vi "hamamatsuReadSegment.vi"() -> ()   [LabVIEW 2017]
uses:
  globalDevices.vi
  globalUtilities.vi
panel:
  out "Frame Count":i32
  out "Numeric":i32
  out "error out":errorcluster {"code" format="%.0x"}
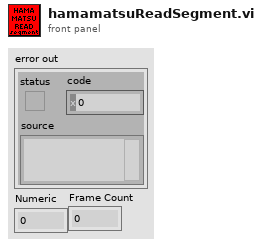
[diagram p1: front panel]
types:
  T1 = enum16{"open", "replace", "create", "open or create", "replace or create", "replace or create with confirmation"}
  T2 = enum16{"big-endian, network order", "native, host order", "little-endian"}
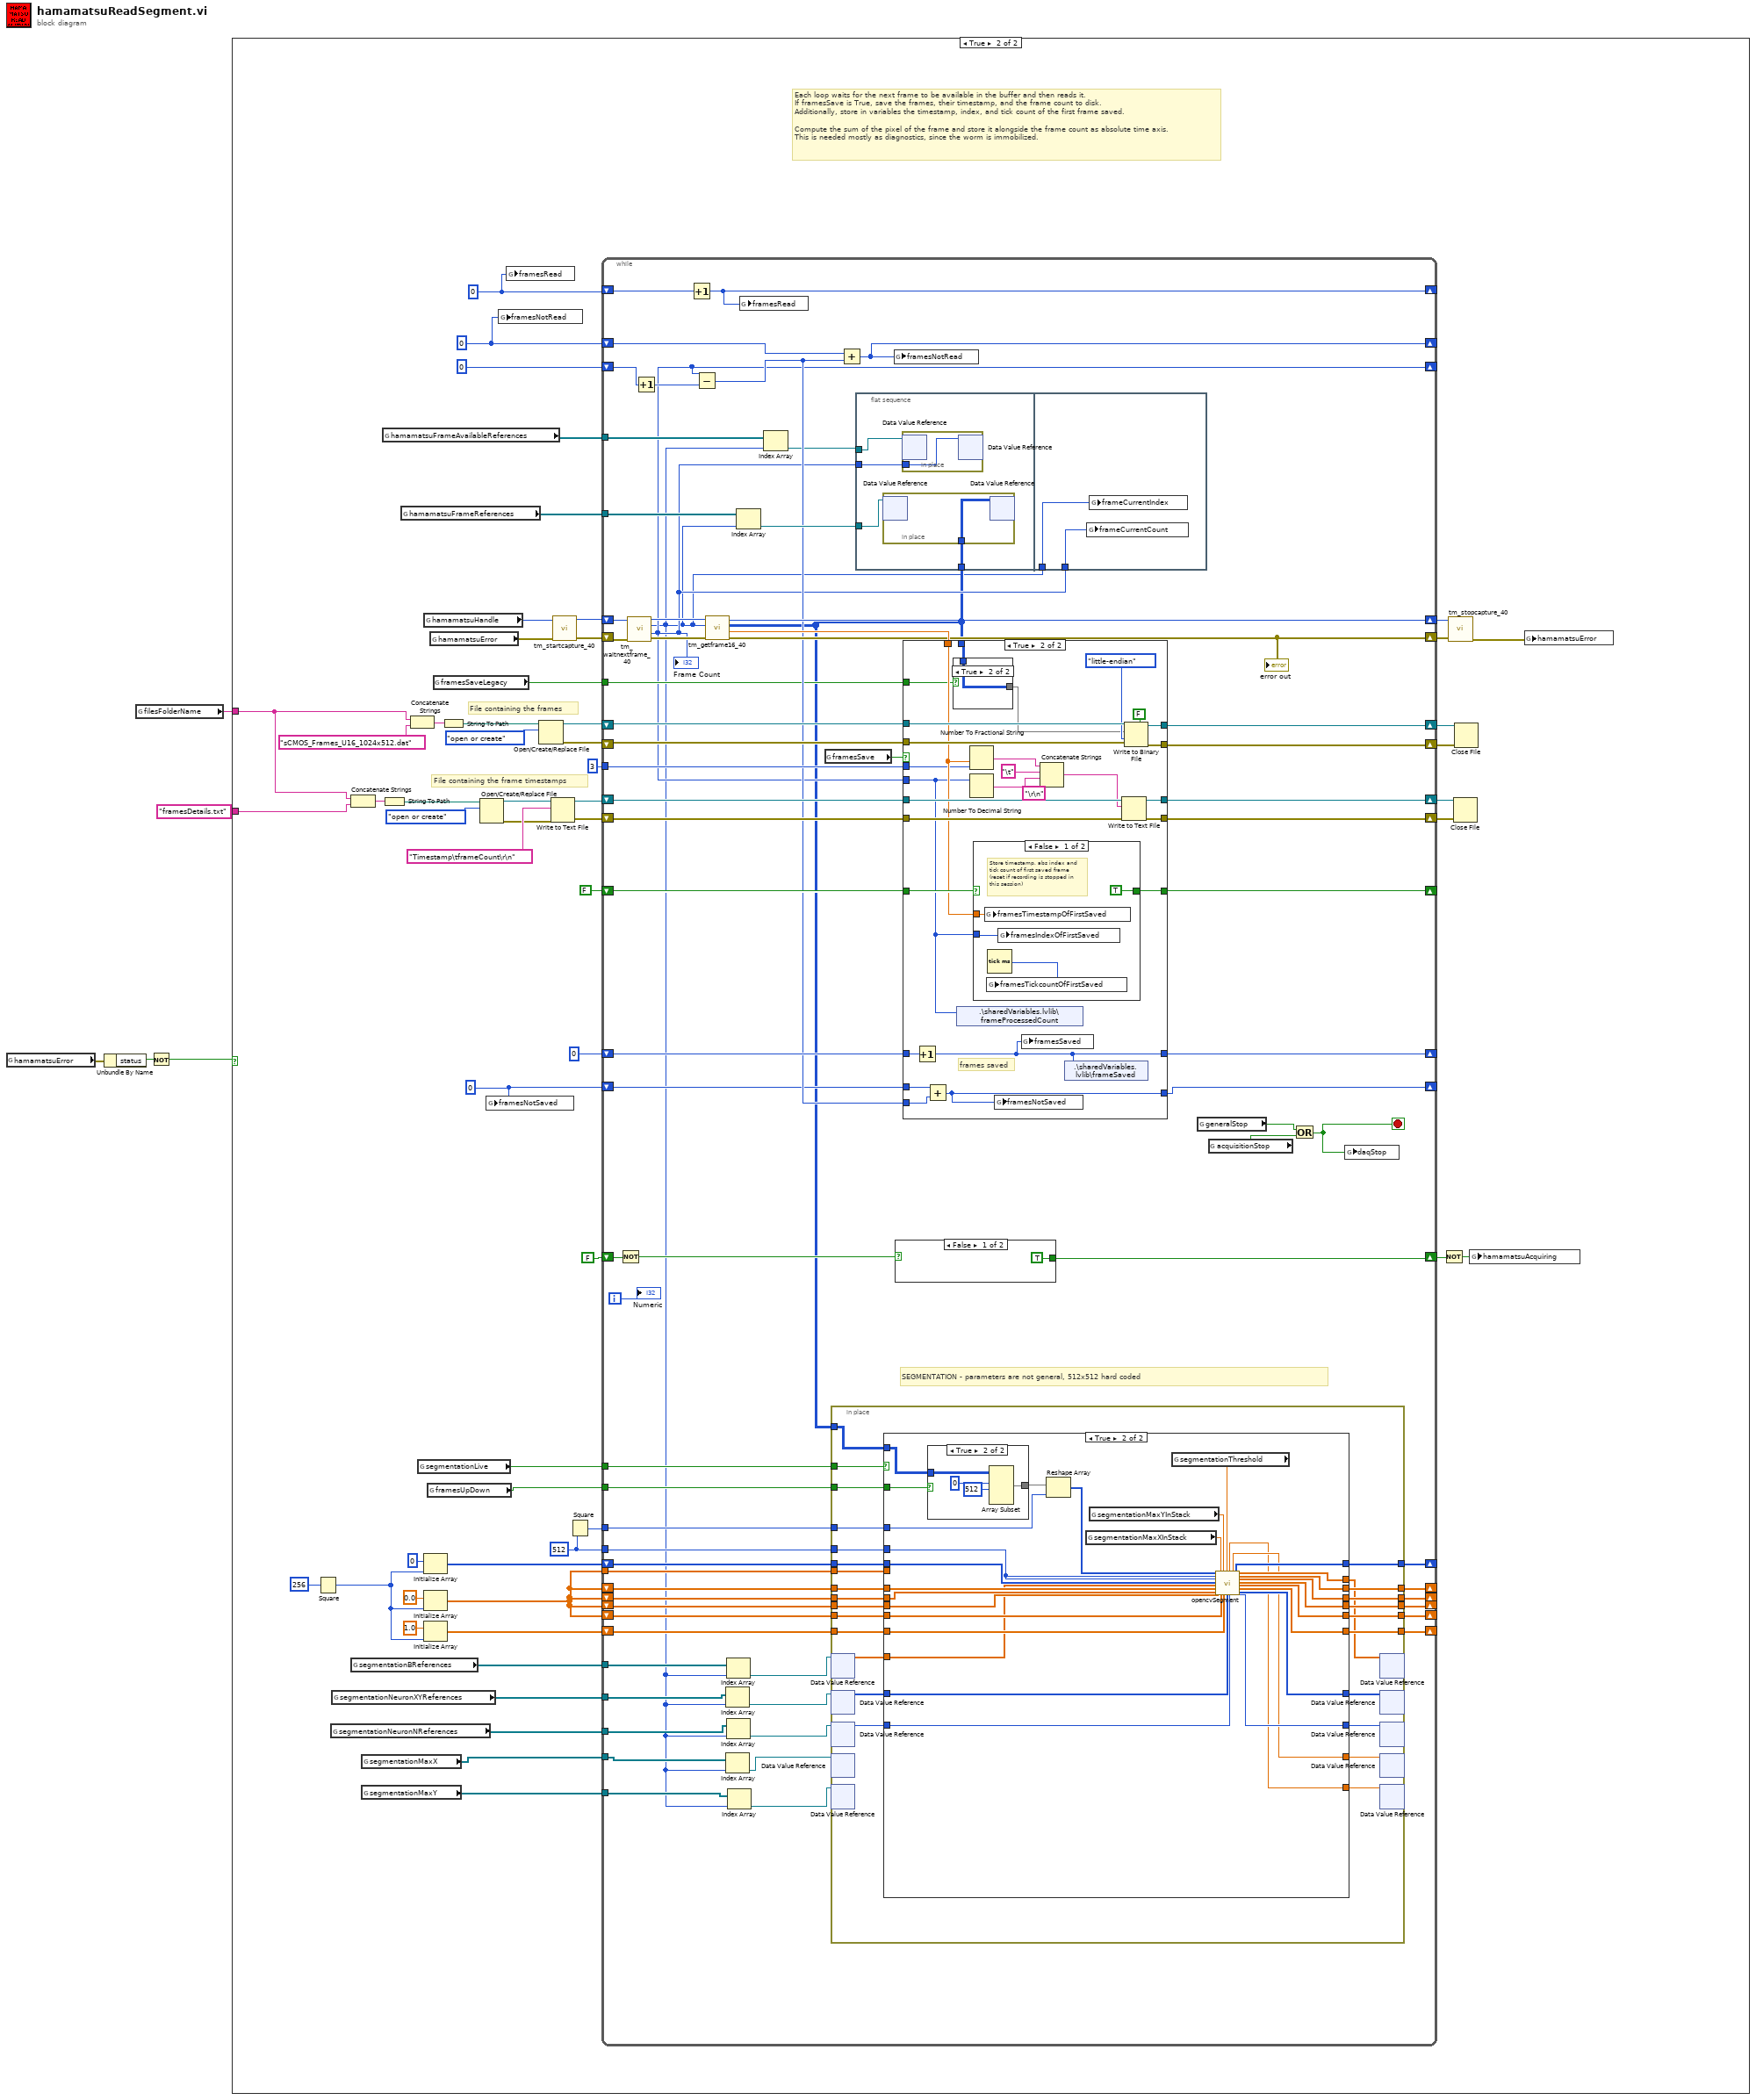
[diagram p0: block diagram]
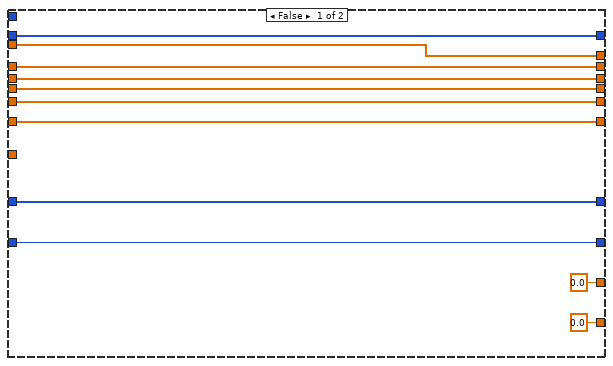
[diagram p3: hidden frame]
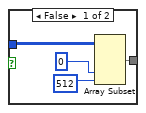
[diagram p4: hidden frame]
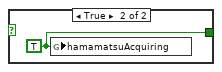
[diagram p5: hidden frame]
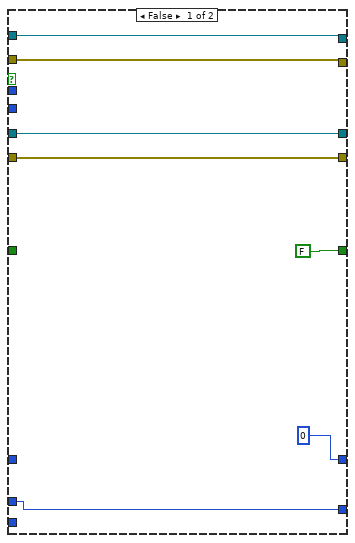
[diagram p6: hidden frame]
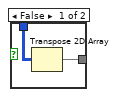
[diagram p7: hidden frame]
diagram:
  n1 = global read "globalDevices.vi" "hamamatsuError"() -> (w3:errorcluster)
  n2 = Unbundle By Name(w3) -> ("status"=w2:bool)
  n3 = global read "globalUtilities.vi" "filesFolderName"() -> (w4:string)
  n4 = Not(x=w2) -> (.not. x?=w1:bool)
  n5 = case shown="True" w1 {
    tunnel: "framesDetails.txt" -> [_ w54]
    tunnel: w4 -> [_ w45]
    frame False {
    }
    frame True {
      w14 = 512 ("sizey")
      w23 = u32 0 ("framesRead")
      w27 = 0
      w24 = 0
      # "Each loop waits for the next frame to be available in the buffer and then reads it.\nIf framesSave is True, save the frames, their timestamp, and the frame count to disk.\nAdditionally, store in variables the timestamp, index, and tick count of the first frame saved.\n\nCompute the sum of the pixel of the frame and store it alongside the frame count as absolute time axis.\nThis is needed mostly as diagnostics, since the worm is immobilized."
      # "File containing the frame timestamps"
      # "File containing the frames"
      n6 = Square(x=256) -> (x^2=w18:i32)
      n7 = global read "globalUtilities.vi" "segmentationNeuronNReferences"() -> (w8:refnum<data-value>[])
      n8 = global read "globalUtilities.vi" "segmentationNeuronXYReferences"() -> (w9:refnum<data-value>[])
      n9 = Concatenate Strings(w45, w54) -> (w55:string)
      n10 = global read "globalUtilities.vi" "segmentationBReferences"() -> (w10:refnum<data-value>[])
      n11 = global read "globalUtilities.vi" "segmentationMaxX"() -> (w7:refnum<data-value>[])
      n12 = global read "globalUtilities.vi" "segmentationMaxY"() -> (w6:refnum<data-value>[])
      n13 = global read "globalDevices.vi" "hamamatsuFrameAvailableReferences"() -> (w28:refnum<data-value>[])
      n14 = String To Path(string=w55) -> (path=w56:path)
      n15 = global read "globalDevices.vi" "hamamatsuFrameReferences"() -> (w32:refnum<data-value>[])
      n16 = Concatenate Strings(w45, "sCMOS_Frames_U16_1024x512.dat") -> (w60:string)
      n17 = global read "globalUtilities.vi" "segmentationLive"() -> (w17:bool)
      n18 = global read "globalDevices.vi" "hamamatsuHandle"() -> (w41:u32)
      n19 = Initialize Array(u16 0 ("element"), w18) -> (w16:u16[])
      n20 = Initialize Array(sgl 0.0 ("element"), w18) -> (w11:sgl[])
      n21 = Initialize Array(sgl 1.0 ("element"), w18) -> (w12:sgl[])
      n22 = global read "globalUtilities.vi" "framesUpDown"() -> (w15:bool)
      n23 = global read "globalDevices.vi" "hamamatsuError"() -> (w42:errorcluster)
      n24 = global read "globalUtilities.vi" "framesSaveLegacy"() -> (w29:bool)
      n25 = String To Path(string=w60) -> (path=w59:path)
      n26 = Open/Create/Replace File(file path (use dialog)=w56, operation (0:open)=T1."open or create") -> (refnum out=w50:refnum<file>, error out=w48:errorcluster)  [unwired: 4 in, 1 out]
      n27 = global write "globalUtilities.vi" "framesNotSaved"(w27) -> ()
      n28 = global write "globalUtilities.vi" "framesNotRead"(w24) -> ()
      n29 = global write "globalUtilities.vi" "framesRead"(w23) -> ()
      n30 = Open/Create/Replace File(file path (use dialog)=w59, operation (0:open)=T1."open or create") -> (refnum out=w58:refnum<file>, error out=w52:errorcluster)  [unwired: 4 in, 1 out]
      n31 = Write to Text File(file (use dialog)=w50, text="Timestamp\tframeCount\r\n", error in=w48) -> (refnum out=w47:refnum<file>, error out=w46:errorcluster)  [unwired: 1 in, 1 out]
      n32 = call <userlib>:"tm_startcapture_40.vi"("error in (no error)"=w42, "Handle in"=w41) -> ("error out"=w43:errorcluster, "Handle out"=w44:u32)  [unwired: 8 in]
      n33 = Square(x=w14) -> (x^2=w13:i32)
      n34 = while {
        shift-right: [w121] -> _
        shift-left: FALSE -> [w122]
        shift-right: [w127] -> w35
        shift-left: w46 -> [w128]
        shift-right: [w125] -> w37
        shift-left: w52 -> [w126]
        tunnel: i16 3 ("precision (6)") -> [w120]
        shift-right: [w119] -> w40
        shift-left: w43 -> [w133]
        shift-right: [w117] -> _
        shift-left: u32 0 -> [w118]
        shift-right: [w116] -> w39
        shift-left: w44 -> [w134]
        shift-right: [w114] -> w34
        shift-left: w47 -> [w129]
        shift-right: [w115] -> w36
        shift-left: w58 -> [w130]
        tunnel: w32 -> [w110]
        shift-right: [w95] -> _
        shift-left: 0 -> [w108]
        shift-right: [w106] -> _
        shift-left: w24 -> [w107]
        shift-right: [w103] -> _
        shift-left: w27 -> [w104]
        tunnel: w29 -> [w102]
        tunnel: w28 -> [w100]
        shift-right: [w97] -> w25
        shift-left: FALSE -> [w99]
        shift-right: [w93] -> _
        shift-left: w23 -> [w94]
        tunnel: w17 -> [w91]
        shift-right: [w85] -> _
        shift-left: w16 -> [w90]
        tunnel: w14 -> [w89]
        tunnel: w15 -> [w87]
        tunnel: w13 -> [w86]
        shift-right: [w79] -> _
        shift-left: w11 -> [w84]
        shift-right: [w78] -> _
        shift-left: w11 -> [w83]
        shift-right: [w77] -> _
        shift-left: w11 -> [w82]
        shift-right: [w76] -> _
        shift-left: w11 -> [w81]
        shift-right: [w75] -> _
        shift-left: w12 -> [w80]
        tunnel: w11 -> [w74]
        tunnel: w10 -> [w73]
        tunnel: w9 -> [w72]
        tunnel: w8 -> [w71]
        tunnel: w7 -> [w67]
        tunnel: w6 -> [w66]
        i -> [w92]
        stop <- w111 stop-if-true
        # "SEGMENTATION - parameters are not general, 512x512 hard coded"
        n35 = Not(x=w99) -> (.not. x?=w98:bool)
        n36 = call <userlib>:"tm_waitnextframe_40.vi"("error in (no error)"=w133, "Handle in"=w134) -> ("error out"=w132:errorcluster, "Frame Count"=w95:i32, "Frame Index"=w63:i32, "Handle out"=w131:u32)  [unwired: 6 in]
        "Frame Count" <- w95
        n37 = Increment(x=w108) -> (x+1=w101:i32)
        n38 = Increment(x=w94) -> (x+1=w93:u32)
        n39 = Subtract(x=w95, y=w101) -> (x-y=w105:i32)
        n40 = call <userlib>:"tm_getframe16_40.vi"("error in (no error)"=w132, "Frame Index"=w63, "Handle in"=w131) -> ("error out"=w119:errorcluster, "Timestamp"=w123:dbl, "Data"=w88:u16[][], "Handle out"=w116:u32)  [unwired: 5 in]
        "error out" <- w119
        n41 = Index Array(array=w72, index=w63) -> (element=w69:refnum<data-value>)
        n42 = Index Array(array=w67, index=w63) -> (element=w64:refnum<data-value>)
        n43 = Index Array(array=w73, index=w63) -> (element=w70:refnum<data-value>)
        n44 = Index Array(array=w71, index=w63) -> (element=w68:refnum<data-value>)
        n45 = Index Array(array=w66, index=w63) -> (element=w65:refnum<data-value>)
        n46 = Index Array(array=w110, index=w63) -> (element=w109:refnum<data-value>)
        n47 = global write "globalUtilities.vi" "framesRead"(w93) -> ()
        n48 = Index Array(array=w100, index=w63) -> (element=w96:refnum<data-value>)
        n49 = global read "globalUtilities.vi" "framesSave"() -> (w124:bool)
        n50 = in-place {
          in-place-border: w91 -> [w160]
          in-place-border: w90 -> [w159]
          in-place-border: w89 -> [w158]
          in-place-border: w88 -> [w157]
          in-place-border: w87 -> [w156]
          in-place-border: w86 -> [w155]
          in-place-border: [w154] -> w85
          in-place-border: w84 -> [w153]
          in-place-border: w83 -> [w152]
          in-place-border: w82 -> [w151]
          in-place-border: w81 -> [w150]
          in-place-border: w80 -> [w149]
          in-place-border: [w148] -> w79
          in-place-border: [w147] -> w78
          in-place-border: [w146] -> w77
          in-place-border: [w145] -> w76
          in-place-border: [w144] -> w75
          in-place-border: w74 -> [w143]
          n51 = in-place-dvr #1(w70) -> (w142:sgl[])  [unwired: 1 out]
          n52 = in-place-dvr #2(w69) -> (w140:u16[])  [unwired: 1 out]
          n53 = in-place-dvr #3(w68) -> (w138:u16)  [unwired: 1 out]
          n54 = in-place-dvr #4(w64) -> ()  [unwired: 2 out]
          n55 = in-place-dvr #5(w65) -> ()  [unwired: 2 out]
          n56 = case shown="True" w160 {
            tunnel: w159 -> [w171 w200]
            tunnel: w158 -> [_ w199]
            tunnel: w157 -> [_ w198]
            tunnel: w156 -> [_ w197]
            tunnel: w155 -> [_ w195]
            tunnel: [w171 w192] -> w154
            tunnel: w153 -> [w170 w191]
            tunnel: w152 -> [w169 w190]
            tunnel: w151 -> [w168 w189]
            tunnel: w150 -> [w167 w188]
            tunnel: w149 -> [w166 w187]
            tunnel: [w165 w186] -> w141
            tunnel: [w170 w185] -> w148
            tunnel: [w169 w184] -> w147
            tunnel: [w168 w183] -> w146
            tunnel: [w167 w182] -> w145
            tunnel: [w166 w181] -> w144
            tunnel: w143 -> [w165 _]
            tunnel: w142 -> [_ w180]
            tunnel: w140 -> [w164 w179]
            tunnel: [w164 w178] -> w139
            tunnel: w138 -> [w163 w177]
            tunnel: [w163 w176] -> w137
            tunnel: [0.0 ("maxX") w175] -> w136
            tunnel: [0.0 ("maxY") w174] -> w135
            frame False {
            }
            frame True {
              n57 = case shown="True" w197 {
                tunnel: w198 -> [w204 w208]
                tunnel: [w201 w205] -> w196
                frame False {
                  n58 = Array Subset(array=w204, index (col)=0 ("index"), length (col)=512 ("length")) -> (w201:u16[][])  [unwired: 2 in]
                }
                frame True {
                  n59 = Array Subset(array=w208, index (row)=0 ("index"), length (row)=512 ("length")) -> (w205:u16[][])  [unwired: 2 in]
                }
              }
              n60 = Reshape Array(w196, w195) -> (w194:u16[])
              n61 = global read "globalUtilities.vi" "segmentationMaxXInStack"() -> (w173:dbl)
              n62 = global read "globalUtilities.vi" "segmentationMaxYInStack"() -> (w172:dbl)
              n63 = global read "globalUtilities.vi" "segmentationThreshold"() -> (w193:sgl)
              n64 = call "opencvSegment.vi"("ImgIn"=w194, "sizex"=w199, "sizey"=w199, "ArrA"=w200, "ArrB"=w180, "ArrBX"=w191, "ArrBY"=w190, "ArrBth"=w189, "maxXInStack"=w173, "ArrBdil"=w188, "maxYInStack"=w172, "ArrUno"=w187, "threshold"=w193, "NeuronXY"=w179, "NeuronN"=w177) -> ("maxY"=w174:dbl, "maxX"=w175:dbl, "ArrA Out"=w192:u16[], "ArrB Out"=w186:sgl[], "ArrBX Out"=w185:sgl[], "ArrBY Out"=w184:sgl[], "ArrBth Out"=w183:sgl[], "ArrBdil Out"=w182:sgl[], "ArrUno Out"=w181:sgl[], "NeuronXY Out"=w178:u16[], "NeuronN Out"=w176:u16)  [unwired: 2 in]
            }
          }
          n65 = in-place-dvr #1(w141) -> ()  [unwired: 2 out]
          n66 = in-place-dvr #2(w139) -> ()  [unwired: 2 out]
          n67 = in-place-dvr #3(w137) -> ()  [unwired: 2 out]
          n68 = in-place-dvr #4(w136) -> ()  [unwired: 2 out]
          n69 = in-place-dvr #5(w135) -> ()  [unwired: 2 out]
        }
        n70 = Add(x=w107, y=w105) -> (x+y=w106:i32)
        n71 = flat-sequence {
          tunnel: w109 -> [w214]
          tunnel: w88 -> [w213]
          tunnel: w96 -> [w212]
          tunnel: w95 -> [w211]
          tunnel: w63 -> [w218]
          tunnel: w95 -> [w217]
          frame #0 {
            n72 = in-place {
              in-place-border: w213 -> [w216]
              n73 = in-place-dvr #6(w214) -> ()  [unwired: 2 out]
              n74 = in-place-dvr #6(w216) -> ()  [unwired: 2 out]
            }
            n75 = in-place {
              in-place-border: w211 -> [w215]
              n76 = in-place-dvr #7(w212) -> ()  [unwired: 2 out]
              n77 = in-place-dvr #7(w215) -> ()  [unwired: 2 out]
            }
          }
          frame #1 {
            n78 = global write "globalUtilities.vi" "frameCurrentCount"(w217) -> ()
            n79 = global write "globalUtilities.vi" "frameCurrentIndex"(w218) -> ()
          }
        }
        n80 = global write "globalUtilities.vi" "framesNotRead"(w106) -> ()
        n81 = case shown="False" w98 {
          tunnel: [TRUE w210] -> w97
          frame False {
          }
          frame True {
            w210 = TRUE ("hamamatsuAcquiring")
            n82 = global write "globalUtilities.vi" "hamamatsuAcquiring"(w210) -> ()
          }
        }
        n83 = case shown="True" w124 {
          tunnel: w130 -> [w221 w253]
          tunnel: w88 -> [_ w229]
          tunnel: w129 -> [w220 w250]
          tunnel: w123 -> [_ w243]
          tunnel: w128 -> [w224 w249]
          tunnel: [w224 w248] -> w127
          tunnel: w126 -> [w225 w247]
          tunnel: [w225 w246] -> w125
          tunnel: w122 -> [_ w245]
          tunnel: [FALSE w244] -> w121
          tunnel: w95 -> [_ w234]
          tunnel: w120 -> [_ w242]
          tunnel: w118 -> [_ w237]
          tunnel: [u32 0 w226] -> w117
          tunnel: [w221 w236] -> w115
          tunnel: [w220 w235] -> w114
          tunnel: w105 -> [_ w232]
          tunnel: w104 -> [w219 w233]
          tunnel: [w219 w231] -> w103
          tunnel: w102 -> [_ w230]
          frame False {
          }
          frame True {
            # "frames saved"
            n84 = Increment(x=w237) -> (x+1=w226:u32)
            n85 = Add(x=w233, y=w232) -> (x+y=w231:i32)
            n86 = case shown="True" w230 {
              tunnel: w229 -> [w255 w256]
              tunnel: [w254 w256] -> w227
              frame False {
                n87 = Transpose 2D Array(2D array=w255) -> (transposed array=w254:u16[][])
              }
              frame True {
              }
            }
            n88 = shared-variable ".\\sharedVariables.lvlib\\frameProcessedCount"(w234) -> ()  [unwired: 1 in, 1 out]
            n89 = Number To Fractional String(number=w243, precision (6)=w242) -> (F-format string=w240:string)  [unwired: 2 in]
            n90 = Number To Decimal String(number=w234) -> (decimal integer string=w239:string)  [unwired: 1 in]
            n91 = case shown="False" w245 {
              selector: w245 -> [_ w261]
              tunnel: [TRUE w261] -> w244
              tunnel: w243 -> [w259 _]
              tunnel: w234 -> [w258 _]
              frame False {
                # "Store timestamp, abs index and\ntick count of first saved frame\n(reset if recording is stopped in\nthis session)"
                n92 = global write "globalUtilities.vi" "framesTimestampOfFirstSaved"(w259) -> ()
                n93 = Tick Count (ms)() -> (millisecond timer value=w257:u32)
                n94 = global write "globalUtilities.vi" "framesTickcountOfFirstSaved"(w257) -> ()
                n95 = global write "globalUtilities.vi" "framesIndexOfFirstSaved"(w258) -> ()
              }
              frame True {
              }
            }
            n96 = global write "globalUtilities.vi" "framesNotSaved"(w231) -> ()
            n97 = global write "globalUtilities.vi" "framesSaved"(w226) -> ()
            n98 = Concatenate Strings(w240, "\t", w239, "\r\n" ("string")) -> (w238:string)
            n99 = shared-variable ".\\sharedVariables.lvlib\\frameSaved"(w226) -> ()  [unwired: 1 in, 1 out]
            n100 = Write to Text File(file (use dialog)=w250, text=w238, error in=w249) -> (refnum out=w235:refnum<file>, error out=w248:errorcluster)  [unwired: 1 in, 1 out]
            n101 = Write to Binary File(file (use dialog)=w253, data=w227, error in=w247, 5:FALSE ("prepend array or string size? (T)"), 9:T2."little-endian" ("byte order (0:big-endian, network order)")) -> (refnum out=w236:refnum<file>, error out=w246:errorcluster)  [unwired: 1 in, 1 out]
          }
        }
        n102 = global read "globalUtilities.vi" "generalStop"() -> (w113:bool)
        n103 = global read "globalUtilities.vi" "acquisitionStop"() -> (w112:bool)
        n104 = Or(x=w113, y=w112) -> (x .or. y?=w111:bool)
        n105 = global write "globalUtilities.vi" "daqStop"(w111) -> ()
        "Numeric" <- w92
      }
      n106 = Not(x=w25) -> (.not. x?=w33:bool)
      n107 = call <userlib>:"tm_stopcapture_40.vi"("error in (no error)"=w40, "Handle in"=w39) -> ("error out"=w38:errorcluster)  [unwired: 8 in, 1 out]
      n108 = Close File(refnum=w34, error in=w35) -> ()  [unwired: 2 out]
      n109 = Close File(refnum=w36, error in=w37) -> ()  [unwired: 2 out]
      n110 = global write "globalUtilities.vi" "hamamatsuAcquiring"(w33) -> ()
      n111 = global write "globalDevices.vi" "hamamatsuError"(w38) -> ()
    }
  }
